vi "Tracking.vi"() -> ()   [LabVIEW 2016]
uses:
  <vilib>/userdefined/High Color/IMAQdx.ctl
  <vilib>/vision/driver/NI_Vision_Acquisition_Software.lvlib
  <vilib>/vision/NI_Vision_Development_Module.lvlib
panel:
  out "Matches[0].Position.y":sgl
  out "Matches[0].Position.x":sgl
  in  "reconnaitre":bool
  in  "stop":bool
  in  "Camera":T1
  out "image":T2(plugin-control)
  out "échantillon":T2(plugin-control)
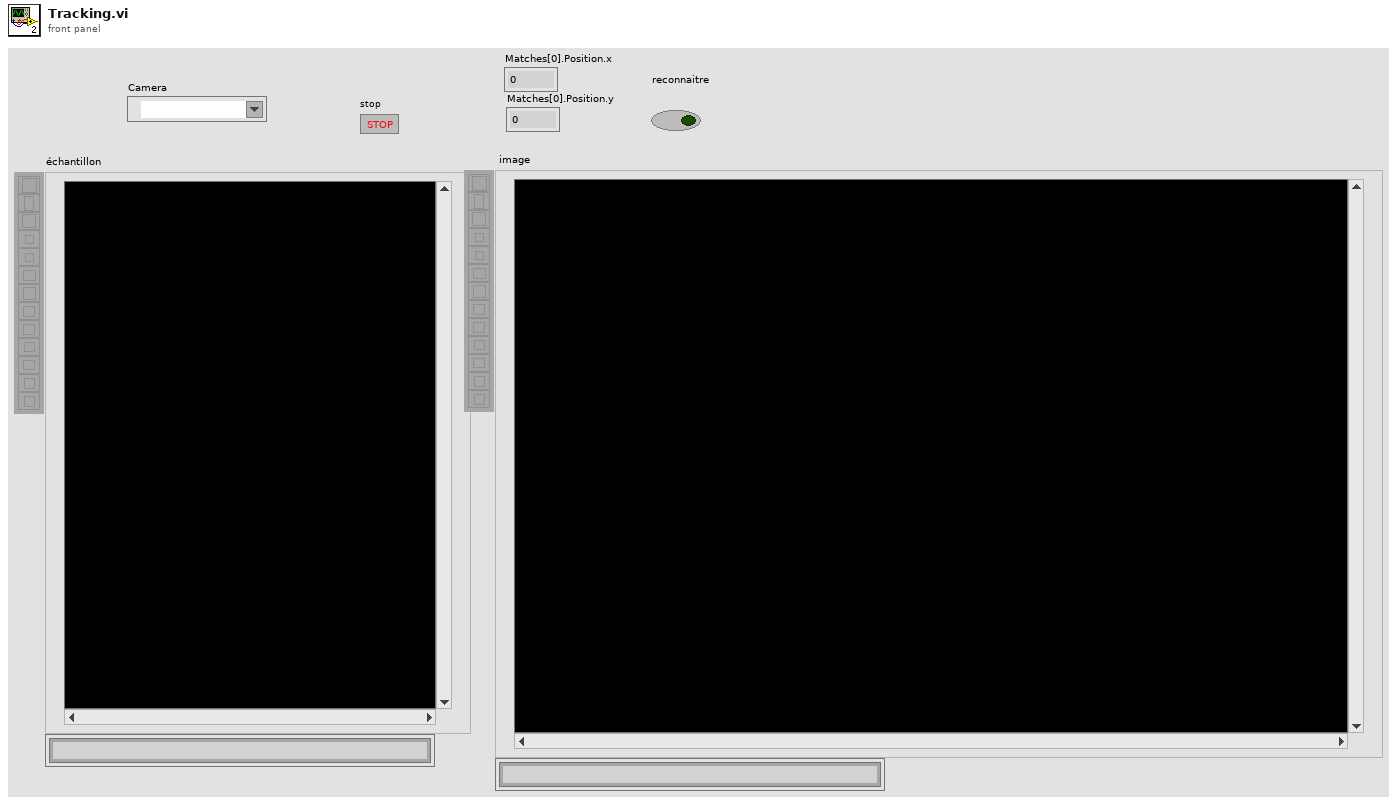
[diagram p1: front panel]
types:
  T1 = typedef "IMAQdx.ctl" = refnum<k21>
  T2 = typedef "IMAQ Image.ctl" = refnum<image>
  T3 = typedef "Image Type" = u32
  T4 = cluster{"Match Mode":u16, "Number of Matches Requested":i32, "Minimum Match Score":sgl, "SubPixel Accuracy":bool, "Rotation Angle Ranges":cluster{"Start":sgl, "End":sgl}[], "Show Search Area":bool, "Show Result":bool}
  T5 = cluster{"Position":cluster{"x":sgl, "y":sgl}, "Angle":sgl, "Scale":sgl, "Score":sgl, "Bounding Box":cluster{"x":sgl, "y":sgl}[]}[]
  T6 = cluster{"Matches[0]":cluster{"Position":cluster{"x":sgl, "y":sgl}, "Angle":sgl, "Scale":sgl, "Score":sgl, "Bounding Box":cluster{"x":sgl, "y":sgl}[]}, "Matches[1]":cluster{"Position":cluster{"x":sgl, "y":sgl}, "Angle":sgl, "Scale":sgl, "Score":sgl, "Bounding Box":cluster{"x":sgl, "y":sgl}[]}, "Matches[2]":cluster{"Position":cluster{"x":sgl, "y":sgl}, "Angle":sgl, "Scale":sgl, "Score":sgl, "Bounding Box":cluster{"x":sgl, "y":sgl}[]}, "Matches[3]":cluster{"Position":cluster{"x":sgl, "y":sgl}, "Angle":sgl, "Scale":sgl, "Score":sgl, "Bounding Box":cluster{"x":sgl, "y":sgl}[]}, "Matches[4]":cluster{"Position":cluster{"x":sgl, "y":sgl}, "Angle":sgl, "Scale":sgl, "Score":sgl, "Bounding Box":cluster{"x":sgl, "y":sgl}[]}, "Matches[5]":cluster{"Position":cluster{"x":sgl, "y":sgl}, "Angle":sgl, "Scale":sgl, "Score":sgl, "Bounding Box":cluster{"x":sgl, "y":sgl}[]}, "Matches[6]":cluster{"Position":cluster{"x":sgl, "y":sgl}, "Angle":sgl, "Scale":sgl, "Score":sgl, "Bounding Box":cluster{"x":sgl, "y":sgl}[]}, "Matches[7]":cluster{"Position":cluster{"x":sgl, "y":sgl}, "Angle":sgl, "Scale":sgl, "Score":sgl, "Bounding Box":cluster{"x":sgl, "y":sgl}[]}, "Matches[8]":cluster{"Position":cluster{"x":sgl, "y":sgl}, "Angle":sgl, "Scale":sgl, "Score":sgl, "Bounding Box":cluster{"x":sgl, "y":sgl}[]}}
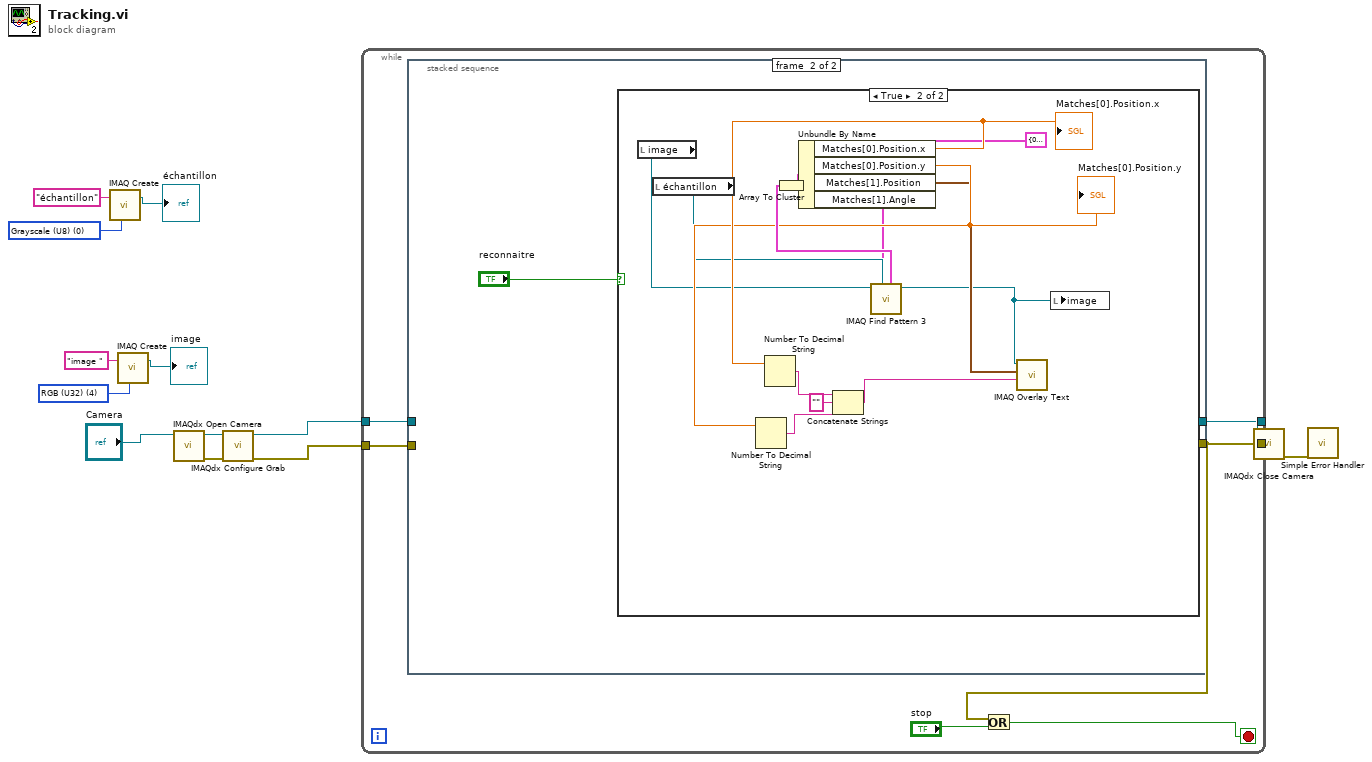
[diagram p0: block diagram]
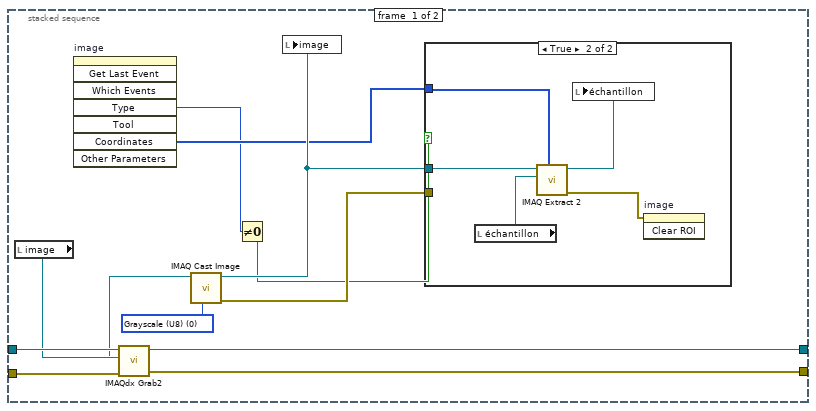
[diagram p2: hidden frame]
diagram:
  w10 = T3 4 items=["Grayscale (U8)", "Grayscale (I16)", "Grayscale (SGL)", "Complex (CSG)", "RGB (U32)", "HSL (U32)", "RGB (U64)", "Grayscale (U16)"] ("Image Type")
  w13 = T3 0 items=["Grayscale (U8)", "Grayscale (I16)", "Grayscale (SGL)", "Complex (CSG)", "RGB (U32)", "HSL (U32)", "RGB (U64)", "Grayscale (U16)"] ("Image Type")
  n1 = call "IMAQ Create"("Image Name"="échantillon", "Image Type"=w13) -> ("New Image"=→"échantillon":T2)  [unwired: 3 in, 1 out]
  n2 = call "IMAQ Create"("Image Name"="image ", "Image Type"=w10) -> ("New Image"=→"image":T2)  [unwired: 3 in, 1 out]
  n3 = call <vilib>:"IMAQdx Open Camera.vi"("Session In"="Camera") -> ("error out"=w6:errorcluster, "Session Out"=w7:T1)  [unwired: 9 in]
  n4 = call <vilib>:"IMAQdx Configure Grab.vi"("error in"=w6, "Session In"=w7) -> ("error out"=w4:errorcluster, "Session Out"=w5:T1)  [unwired: 8 in]
  n5 = while {
    tunnel: w5 -> [w20]
    tunnel: w4 -> [w19]
    tunnel: [w17] -> w3
    tunnel: [w18] -> w2
    stop <- w15 stop-if-true
    n6 = stacked-sequence {
      tunnel: w20 -> [w32 _]
      tunnel: w19 -> [w23 _]
      tunnel: [w22 _] -> w17
      tunnel: [w21 _] -> w18
      frame #0 {
        w29 = T3 0 items=["Grayscale (U8)", "Grayscale (I16)", "Grayscale (SGL)", "Complex (CSG)", "RGB (U32)", "HSL (U32)", "RGB (U64)", "Grayscale (U16)"] ("Image Type")
        n7 = local read "image"() -> (w31:T2)
        n8 = invoke on="image" class="ImageControl" method="Get Last Event"() -> ("Type"=w25:i32, "Coordinates"=w26:i32[])  [unwired: 8 in, 6 out]
        n9 = call <vilib>:"IMAQdx Grab2.vi"("error in"=w23, "Image In"=w31, "Session In"=w32) -> ("error out"=w22:errorcluster, "Image Out"=w30:T2, "Session Out"=w21:T1)  [unwired: 5 in, 1 out]
        n10 = call "IMAQ Cast Image"("Image Type"=w29, "Image Src"=w30) -> ("error out"=w28:errorcluster, "Image Dst Out"=w27:T2)  [unwired: 8 in]
        n11 = Not Equal To 0?(x=w25) -> (x != 0?=w24:bool)
        n12 = local write "image"(w27) -> ()
        n13 = case shown="True" w24 {
          tunnel: w27 -> [_ w37]
          tunnel: w28 -> [_ _]
          tunnel: w26 -> [_ w34]
          frame False {
          }
          frame True {
            n14 = local read "échantillon"() -> (w36:T2)
            n15 = call "IMAQ Extract 2"("Optional Rectangle"=w34, "Image Dst"=w36, "Image Src"=w37) -> ("error out"=w33:errorcluster, "Image Dst Out"=w35:T2)  [unwired: 7 in]
            n16 = local write "échantillon"(w35) -> ()
            n17 = invoke on="image" class="ImageControl" method="Clear ROI"(error in=w33) -> ()  [unwired: 2 in, 3 out]
          }
        }
      }
      frame #1 {
        n18 = case shown="True" "reconnaitre" {
          frame False {
          }
          frame True {
            n19 = local read "image"() -> (w41:T2)
            n20 = local read "échantillon"() -> (w40:T2)
            n21 = call "IMAQ Find Pattern 3"("Settings"=T4 {"Match Mode"=0, "Number of Matches Requested"=1, "Minimum Match Score"=800.0, "SubPixel Accuracy"=FALSE, "Rotation Angle Ranges"=[], "Show Search Area"=FALSE, "Show Result"=TRUE}, "Template"=w40, "Image"=w41) -> ("Image Out"=w42:T2, "Matches"=w51:T5)  [unwired: 3 in, 4 out]
            n22 = Array To Cluster(array=w51) -> (cluster=w50:T6)
            n23 = Unbundle By Name(w50) -> ("Matches[0].Position.x"=w47:sgl, "Matches[0].Position.y"=w46:sgl, "Matches[1].Position"=w43:cluster{"x":sgl, "y":sgl})  [unwired: 1 out]
            "Matches[0].Position.x" <- w47
            "Matches[0].Position.y" <- w46
            n24 = Number To Decimal String(number=w46) -> (decimal integer string=w48:string)  [unwired: 1 in]
            n25 = Number To Decimal String(number=w47) -> (decimal integer string=w49:string)  [unwired: 1 in]
            n26 = Concatenate Strings(w49, "" ("string"), w48) -> (w44:string)
            n27 = call "IMAQ Overlay Text"("String"=w44, "Origin"=w43, "Image"=w42) -> ()  [unwired: 7 in, 2 out]
            n28 = local write "image"(w42) -> ()
          }
        }
      }
    }
    n29 = Or(x=w17, y="stop") -> (x .or. y?=w15:bool)
  }
  n30 = call <vilib>:"IMAQdx Close Camera.vi"("error in"=w3, "Session In"=w2) -> ("error out"=w1:errorcluster)  [unwired: 9 in]
  n31 = call <vilib>:"Simple Error Handler.vi"("error in (no error)"=w1) -> ()  [unwired: 4 in, 5 out]
